vi "CollisionAvoidance_main.vi"(8 "Error In":errorcluster) -> (0 "Error Out":errorcluster)   [LabVIEW 2013]
uses:
  My Computer/Controls/Steering Inputs.ctl
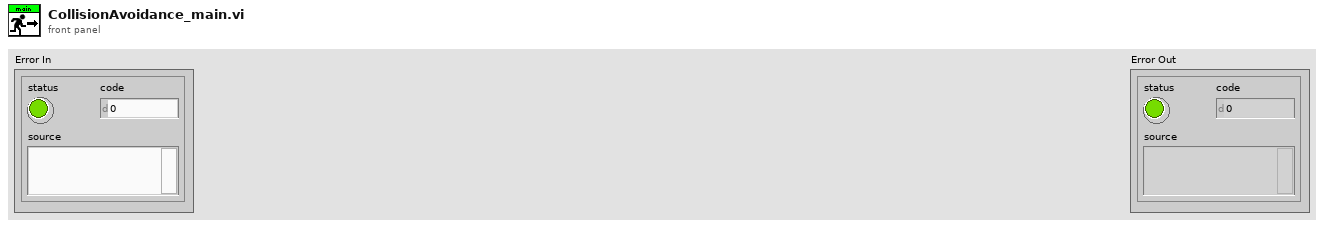
[diagram p1: front panel]
types:
  T1 = typedef "Steering Inputs.ctl" = cluster{"X":dbl, "Y":dbl, "Z":dbl, "phi":dbl, "theta":dbl, "psi":dbl}
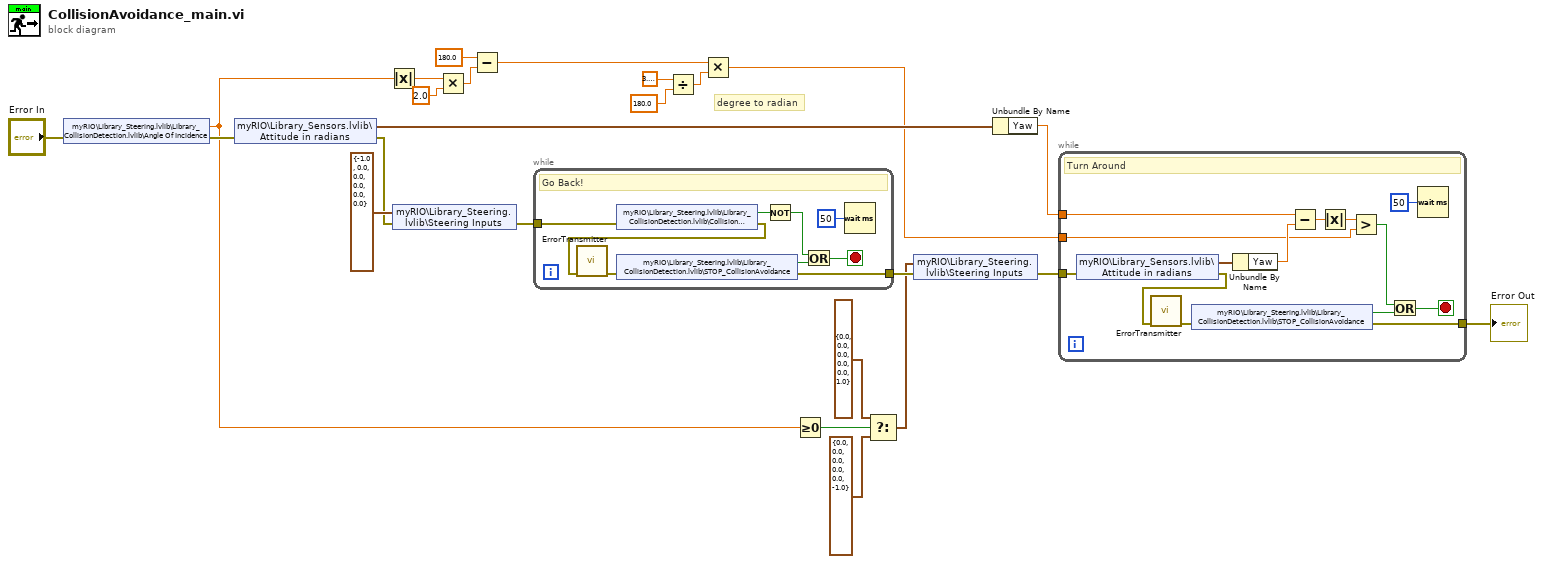
[diagram p0: block diagram]
diagram:
  # "degree to radian"
  n1 = shared-variable "myRIO\\Library_Steering.lvlib\\Library_CollisionDetection.lvlib\\Angle Of Incidence"(error in="Error In") -> (w8:dbl, error out=w15:errorcluster)
  n2 = shared-variable "myRIO\\Library_Sensors.lvlib\\Attitude in radians"(error in=w15) -> (w18:cluster{"Roll":dbl, "Pitch":dbl, "Yaw":dbl}, error out=w19:errorcluster)
  n3 = Absolute Value(x=w8) -> (abs(x)=w7:dbl)
  n4 = shared-variable "myRIO\\Library_Steering.lvlib\\Steering Inputs"(T1 {"X"=-1.0, "Y"=0.0, "Z"=0.0, "phi"=0.0, "theta"=0.0, "psi"=0.0} ("Steering Inputs"), error in=w19) -> (error out=w23:errorcluster)
  n5 = Multiply(x=w7, y=2.0) -> (x*y=w9:dbl)
  n6 = Subtract(x=180.0, y=w9) -> (x-y=w5:dbl)
  n7 = while {
    tunnel: w23 -> [w28]
    tunnel: [w25] -> w22
    stop <- w29 stop-if-true
    # "Go Back!"
    n8 = shared-variable "myRIO\\Library_Steering.lvlib\\Library_CollisionDetection.lvlib\\Collision Detected"(error in=w28) -> (w32:bool, error out=w26:errorcluster)
    n9 = call "ErrorTransmitter.vi"("Error In"=w26) -> ("Error Out"=w27:errorcluster)  [unwired: 10 in]
    n10 = shared-variable "myRIO\\Library_Steering.lvlib\\Library_CollisionDetection.lvlib\\STOP_CollisionAvoidance"(error in=w27) -> (w31:bool, error out=w25:errorcluster)
    n11 = Not(x=w32) -> (.not. x?=w30:bool)
    n12 = Or(x=w30, y=w31) -> (x .or. y?=w29:bool)
    n13 = Wait (ms)(milliseconds to wait=u32 50) -> ()  [unwired: 1 out]
  }
  n14 = Divide(x=3.141592653589793, y=180.0) -> (x/y=w4:dbl)
  n15 = Multiply(x=w5, y=w4) -> (x*y=w1:dbl)
  n16 = Greater Or Equal To 0?(x=w8) -> (x >= 0?=w14:bool)
  n17 = Select(t=T1 {"X"=0.0, "Y"=0.0, "Z"=0.0, "phi"=0.0, "theta"=0.0, "psi"=1.0} ("Steering Inputs"), s=w14, f=T1 {"X"=0.0, "Y"=0.0, "Z"=0.0, "phi"=0.0, "theta"=0.0, "psi"=-1.0} ("Steering Inputs")) -> (s? t:f=w11:T1)
  n18 = shared-variable "myRIO\\Library_Steering.lvlib\\Steering Inputs"(w11, error in=w22) -> (error out=w20:errorcluster)
  n19 = Unbundle By Name(w18) -> ("Yaw"=w17:dbl)
  n20 = while {
    tunnel: [w44] -> w21
    tunnel: w20 -> [w41]
    tunnel: w17 -> [w39]
    tunnel: w1 -> [w34]
    stop <- w45 stop-if-true
    # "Turn Around"
    n21 = shared-variable "myRIO\\Library_Sensors.lvlib\\Attitude in radians"(error in=w41) -> (w42:cluster{"Roll":dbl, "Pitch":dbl, "Yaw":dbl}, error out=w35:errorcluster)
    n22 = call "ErrorTransmitter.vi"("Error In"=w35) -> ("Error Out"=w47:errorcluster)  [unwired: 10 in]
    n23 = shared-variable "myRIO\\Library_Steering.lvlib\\Library_CollisionDetection.lvlib\\STOP_CollisionAvoidance"(error in=w47) -> (w43:bool, error out=w44:errorcluster)
    n24 = Unbundle By Name(w42) -> ("Yaw"=w40:dbl)
    n25 = Subtract(x=w39, y=w40) -> (x-y=w38:dbl)
    n26 = Absolute Value(x=w38) -> (abs(x)=w37:dbl)
    n27 = Greater?(x=w37, y=w34) -> (0:w36:bool)
    n28 = Or(x=w36, y=w43) -> (x .or. y?=w45:bool)
    n29 = Wait (ms)(milliseconds to wait=u32 50) -> ()  [unwired: 1 out]
  }
  "Error Out" <- w21
